vi "Main.vi"(11 "Module Admin":refnum<class "Delacor_lib_QMH_Cloneable Module Admin.lvclass">) -> ()   [LabVIEW 2020, in "Arduino stepper.lvlib"]
doc: "This template is based off of the Queued Message Handler design pattern and the Queued Message Handler project template that ships with LabVIEW.\n\nThe main difference is that the queue is private to this module and communication between modules is performed via Broadcast and Request events.\n\nRequest events are wrapped in public API methods and are handled in the Event Handling Loop (EHL) of this VI. Any module can register for Broadcast events sent by this module. The EHL generates messages based on user interface actions.\n\nThe Message Handling Loop (MHL) processes messages generated by the EHL, or by other messages. The messages are string values, so new messages can be added easily to the Message Cases case structure in the MHL. Each message cluster can also provide an optional value for Message Data, which is a variant that can be converted to whatever message-specific data is required.\n_____\nBased on DQMH Project Template 6.1.0.94."
uses:
  Arduino stepper.lvlib
  <vilib>/Delacor/Delacor QMH/Libraries/Cloneable Module Admin_class/Delacor_lib_QMH_Cloneable Module Admin.lvclass
  C:/Program Files (x86)/National Instruments/LabVIEW 2020/vi.lib/Delacor/Delacor QMH/Libraries/Module Admin_class/Delacor_lib_QMH_Module Admin.lvclass
  Module Data--cluster.ctl
  Stop continuous reading Argument--cluster.ctl
  <vilib>/Delacor/Delacor QMH/Libraries/Message Queue_class/Delacor_lib_QMH_Message Queue.lvclass/Delacor_lib_QMH_Message Queue.ctl
  <vilib>/Delacor/Delacor QMH/Libraries/Cloneable Module Admin_class/Delacor_lib_QMH_Cloneable Module Admin.lvclass/Delacor_lib_QMH_Cloneable Module Admin.ctl
  Stop Argument--cluster.ctl
  <vilib>/Delacor/Delacor QMH/Libraries/Module Admin_class/Delacor_lib_QMH_Module Admin.lvclass/Delacor_lib_QMH_Module Admin.ctl
  Connect Argument--cluster.ctl
  Support/COM params--typedef.ctl
  Connect (Reply Payload)--cluster.ctl
  Disconnect Argument--cluster.ctl
  Move motor Argument--cluster.ctl
  Support/Motor parameters.ctl
  Support/Motor direction -- enum.ctl
  Get position Argument--cluster.ctl
  Get position (Reply Payload)--cluster.ctl
  Read port continuously Argument--cluster.ctl
  Stop motor Argument--cluster.ctl
  Read end-stops Argument--cluster.ctl
  Read end-stops (Reply Payload)--cluster.ctl
  Read all info Argument--cluster.ctl
  <vilib>/Utility/miscctls.llb/LVPointTypeDef.ctl
  <vilib>/Instr/_visa.llb/VISA Flush IO Buffer Mask.ctl
  Support/Wake HL args--typedef.ctl
  <vilib>/Delacor/Delacor QMH/Libraries/Message Queue_class/Delacor_lib_QMH_Enqueue Message (Single).vi
  <vilib>/Delacor/Delacor QMH/Libraries/Cloneable Module Admin_class/Delacor_lib_QMH_Get Module ID.vi
  <vilib>/Delacor/Delacor QMH/Libraries/Module Admin_class/Delacor_lib_QMH_Get External Launch.vi
  <vilib>/Utility/error.llb/Error Cluster From Error Code.vi
  <vilib>/ErrorRing/Error Ring.xnode
  <vilib>/Delacor/Delacor QMH/Libraries/Message Queue_class/Delacor_lib_QMH_Message Queue.lvclass
panel:
  out "End-stops":cluster{"ES1":bool, "ES2":bool}
  out "read buffer 2":string
  out "Position":i32
  out "Data read":string
  out "*(type *) &x":string
  out "error out":errorcluster
  out "Status":string
  in  "Simulate EHL Error":bool
  in  "Simulate MHL Error":bool
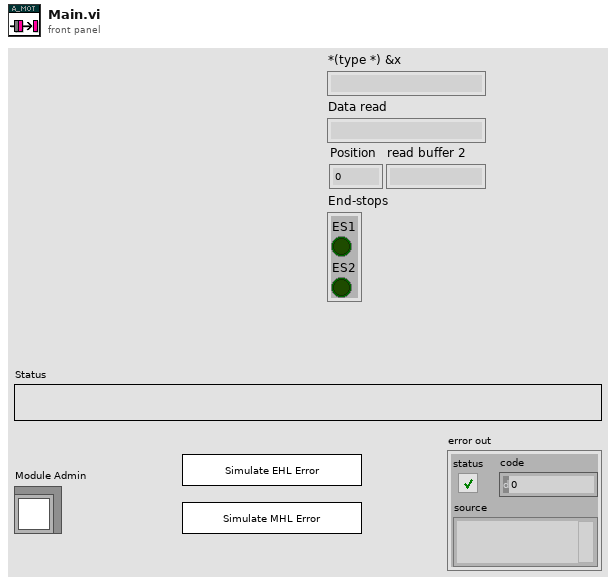
[diagram p1: front panel]
types:
  T1 = typedef "Arduino stepper.lvlib/Request Events--cluster.ctl" = cluster{"Stop Module":refnum<user-event>, "Show Panel":refnum<user-event>, "Hide Panel":refnum<user-event>, "Show Diagram":refnum<user-event>, "Get Module Execution Status":refnum<user-event>, "Connect":refnum<user-event>, "Disconnect":refnum<user-event>, "Move motor":refnum<user-event>, "Get position":refnum<user-event>, "Read port continuously":refnum<user-event>, "Stop continuous reading":refnum<user-event>, "Stop motor":refnum<user-event>, "Read end-stops":refnum<user-event>, "Read all info":refnum<user-event>}
  T2 = cluster{"Wake HL":refnum<user-event>, "Sleep HL":refnum<user-event>}
  T3 = typedef "Arduino stepper.lvlib/Module Data--cluster.ctl" = cluster{"Status":string, "VISA resource":refnum<visa-resource-name>, "Connected?":bool}
  T4 = typedef "Arduino stepper.lvlib/Stop continuous reading Argument--cluster.ctl" = cluster{"Module ID":i32, "Boolean":bool}
  T5 = enum32{"invalid lock state", "Not Locked", "Locked (No Password)", "Password-protected"}
  T6 = typedef "Arduino stepper.lvlib/Stop Argument--cluster.ctl" = cluster{"Module ID":i32, "Origin":string, "Exit via Stop Module Req?":bool, "Wait for Module to stop?":bool}
  T7 = typedef "Arduino stepper.lvlib/Connect Argument--cluster.ctl" = cluster{"Module ID":i32, "VISA resource":refnum<visa-resource-name>, "COM params":T8, "Wait Notifier":refnum<notifier>, "wait for reply":bool}
  T8 = typedef "Arduino stepper.lvlib/COM params--typedef.ctl" = cluster{"baud rate":u32, "data bits":u16, "parity":enum16{"None", "Odd", "Even", "Mark", "Space"}, "stop bits":u16, "flow control":u16}
  T9 = typedef "Arduino stepper.lvlib/Disconnect Argument--cluster.ctl" = cluster{"Module ID":i32, "Boolean":bool}
  T10 = typedef "Arduino stepper.lvlib/Move motor Argument--cluster.ctl" = cluster{"Module ID":i32, "Motor params":T11}
  T11 = typedef "Arduino stepper.lvlib/Motor parameters.ctl" = cluster{"Motor type":enum8{"", "Unipolar", "Bipolar"}, "Direction":T12, "Steps":u16, "Frequency (Hz)":u8, "Step type":enum8{"", "Half", "Full"}}
  T12 = typedef "Arduino stepper.lvlib/Motor direction -- enum.ctl" = enum8{"", "CW", "CCW"}
  T13 = typedef "Arduino stepper.lvlib/Get position Argument--cluster.ctl" = cluster{"Module ID":i32, "Wait Notifier":refnum<notifier>, "wait for reply":bool}
  T14 = typedef "Arduino stepper.lvlib/Read port continuously Argument--cluster.ctl" = cluster{"Module ID":i32, "Timeout":i32}
  T15 = typedef "Arduino stepper.lvlib/Stop motor Argument--cluster.ctl" = cluster{"Module ID":i32, "Boolean":bool}
  T16 = typedef "Arduino stepper.lvlib/Read end-stops Argument--cluster.ctl" = cluster{"Module ID":i32, "Wait Notifier":refnum<notifier>, "wait for reply":bool}
  T17 = typedef "Arduino stepper.lvlib/Read all info Argument--cluster.ctl" = cluster{"Module ID":i32, "Boolean":bool}
  T18 = typedef "LVPointTypeDef.ctl" = cluster{"Horizontal":i16, "Vertical":i16}
  T19 = enum32{"Invalid", "Standard", "Closed", "Hidden", "Minimized", "Maximized"}
  T20 = typedef "Arduino stepper.lvlib/Connect (Reply Payload)--cluster.ctl" = cluster{"error":errorcluster, "Connected?":bool}
  T21 = typedef "Arduino stepper.lvlib/Get position (Reply Payload)--cluster.ctl" = cluster{"Position":i32, "error":errorcluster, "End position?":bool}
  T22 = typedef "Arduino stepper.lvlib/Read end-stops (Reply Payload)--cluster.ctl" = cluster{"End-stops":cluster{"ES1":bool, "ES2":bool}, "error":errorcluster}
  T23 = typedef "Arduino stepper.lvlib/Wake HL args--typedef.ctl" = cluster{"VISA resource name":refnum<visa-resource-name>, "Timeout":i32, "Module ID":i32}
  T24 = typedef "VISA Flush IO Buffer Mask.ctl" = u16
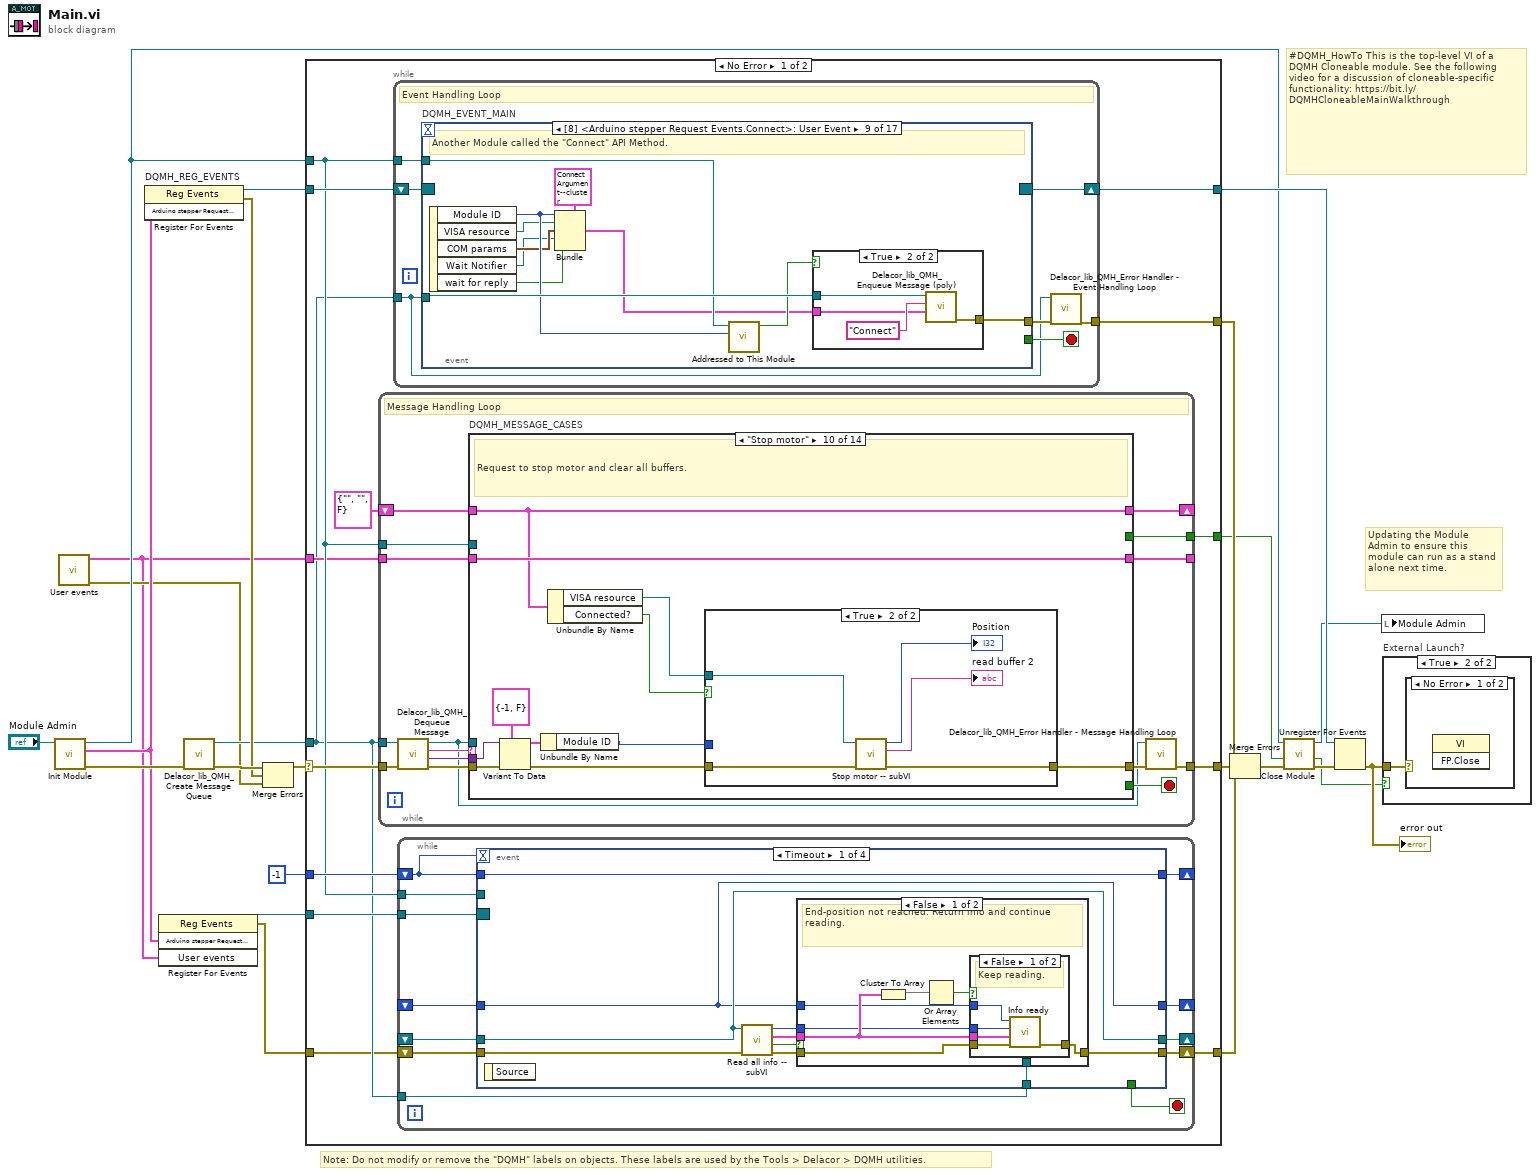
[diagram p0: block diagram]
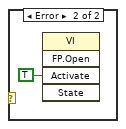
[diagram p3: hidden frame]
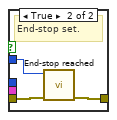
[diagram p4: hidden frame]
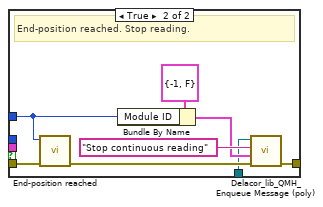
[diagram p5: hidden frame]
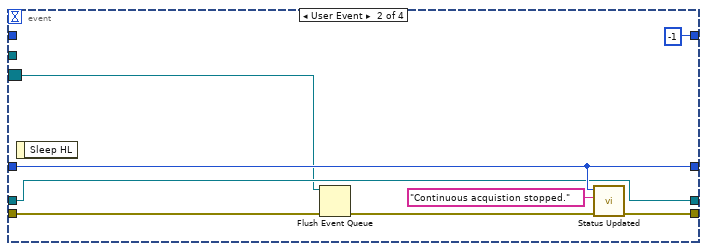
[diagram p6: hidden frame]
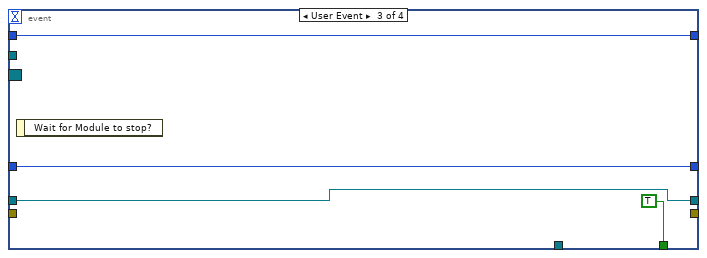
[diagram p7: hidden frame]
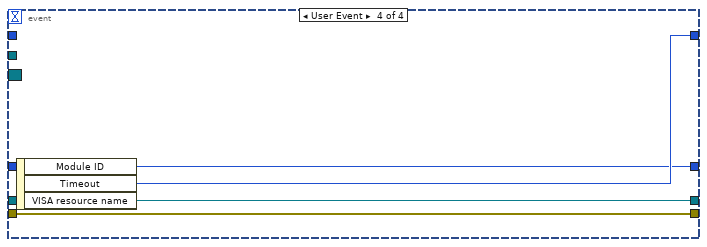
[diagram p8: hidden frame]
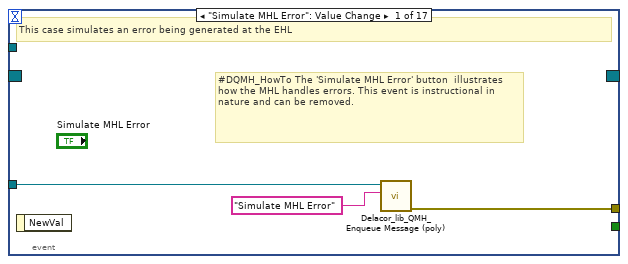
[diagram p9: hidden frame]
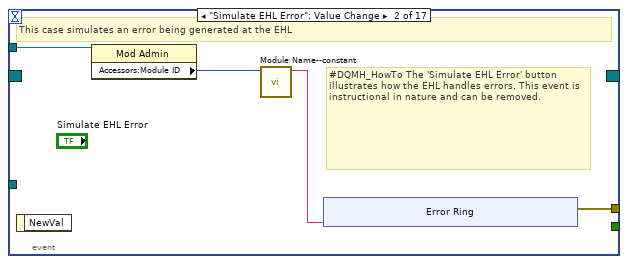
[diagram p10: hidden frame]
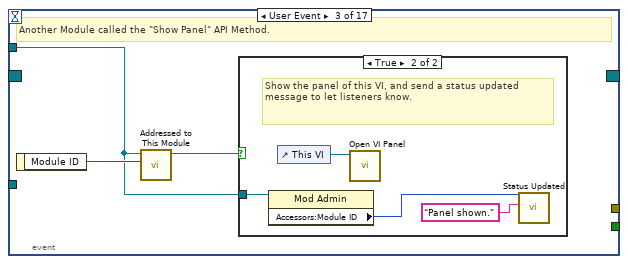
[diagram p11: hidden frame]
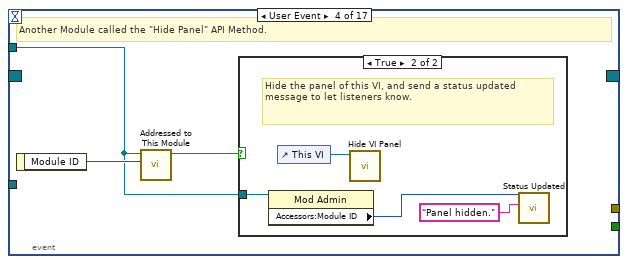
[diagram p13: hidden frame]
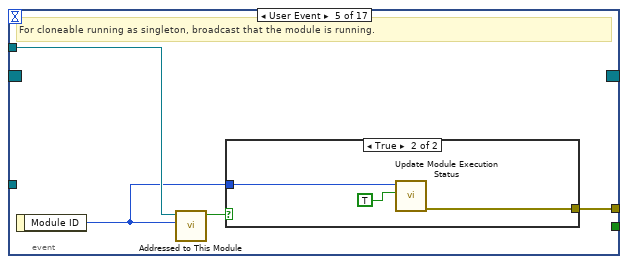
[diagram p15: hidden frame]
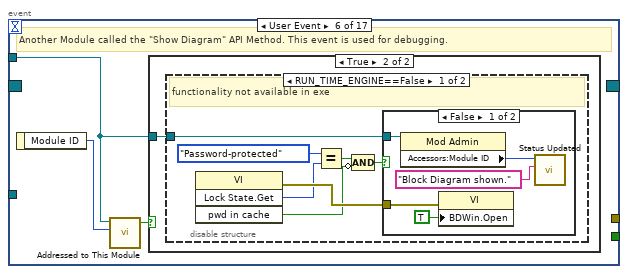
[diagram p17: hidden frame]
diagram:
  # "#DQMH_HowTo This is the top-level VI of a DQMH Cloneable module. See the following video for a discussion of cloneable-specific functionality: https://bit.ly/DQMHCloneableMainWalkthrough"
  # "Note: Do not modify or remove the \"DQMH\" labels on objects. These labels are used by the Tools > Delacor > DQMH utilities."
  # "Updating the Module Admin to ensure this module can run as a stand alone next time."
  n1 = call "Init Module.vi"("Cloneable Module Admin in"="Module Admin") -> ("error out"=w21:errorcluster, "Arduino stepper Request Events"=w8:T1, "Cloneable Module Admin out"=w5:refnum<class "Delacor_lib_QMH_Cloneable Module Admin.lvclass">)  [unwired: 8 in]
  n2 = call "User events.vi"() -> ("error out"=w4:errorcluster, "User events"=w3:T2)  [unwired: 10 in]
  n3 = register-events "DQMH_REG_EVENTS"(w8) -> (reference out=w14:refnum<event-registration>, error out=w16:errorcluster)  [unwired: 2 in]
  n4 = register-events(w8, w3) -> (reference out=w7:refnum<event-registration>, error out=w1:errorcluster)  [unwired: 2 in]
  n5 = call <vilib>:"Delacor_lib_QMH_Create Message Queue.vi"("error in"=w21) -> ("error out"=w18:errorcluster, "Message Queue"=w13:refnum<class "Delacor_lib_QMH_Message Queue.lvclass">)  [unwired: 9 in]
  n6 = Merge Errors(w18, w16, w4) -> (w17:errorcluster)
  n7 = case shown="No Error" w17 {
    selector: w17 -> [w36 w626]
    tunnel: [w38 w625] -> w22
    tunnel: [w35 w633] -> w15
    tunnel: w14 -> [w33 w633]
    tunnel: w13 -> [w27 w624]
    tunnel: [w37 _] -> w23
    tunnel: w5 -> [w29 w629]
    tunnel: [w32 _] -> w10
    tunnel: w7 -> [w31 _]
    tunnel: -1 -> [w30 _]
    tunnel: w3 -> [w28 _]
    tunnel: [w26 w623] -> w2
    tunnel: w1 -> [w25 w623]
    frame No Error {
      n8 = while {
        tunnel: w27 -> [w307]
        shift-right: [w311] -> _
        shift-left: T3 {"Status"="", "VISA resource"="", "Connected?"=FALSE} ("Data Cluster") -> [w312]
        tunnel: w36 -> [w315]
        tunnel: [w313] -> w38
        tunnel: w29 -> [w305]
        tunnel: [w304] -> w32
        tunnel: w28 -> [w303]
        tunnel: [w302] -> _
        stop <- w310 stop-if-true
        # "Message Handling Loop"
        n9 = call-dynamic "Delacor_lib_QMH_Dequeue Message.vi"("error in"=w315, "Message Queue in"=w307) -> ("error out"=w314:errorcluster, "Message Data"=w308:variant, "Message"=w309:string, "Message Queue out"=w306:refnum<class "Delacor_lib_QMH_Message Queue.lvclass">)  [unwired: 6 in]
        n10 = case "DQMH_MESSAGE_CASES" shown="\"Stop motor\"" w309 {
          selector: w309 -> [_ _ _ _ _ _ _ _ _ _ _ _ _ w610]
          tunnel: w306 -> [_ _ _ _ _ _ _ _ _ _ _ w566 w596 _]
          tunnel: w314 -> [w336 w359 w383 w409 w437 w469 w488 w511 w534 w551 w563 w575 w601 w612]
          tunnel: [w334 w351 w376 w403 w428 w460 w479 w507 w526 w543 w563 w571 w599 w613] -> w316
          tunnel: w312 -> [w327 w346 w373 w405 w427 w458 w482 w505 w533 w545 w562 w570 w584 w611]
          tunnel: [w326 w344 w371 w405 w427 w458 w482 w505 w533 w545 w562 w570 w584 w611] -> w311
          tunnel: [_ _ _ _ _ _ _ _ _ _ _ _ w595 _] -> w310
          tunnel: w308 -> [_ w357 w382 w408 w435 w467 w487 w510 w532 w550 _ w569 w593 _]
          tunnel: w305 -> [w321 _ _ _ _ _ _ _ w529 _ _ w568 w589 w608]
          tunnel: [_ _ _ _ _ _ _ _ _ _ _ _ w591 _] -> w304
          tunnel: w303 -> [w317 w347 w377 w402 w423 w459 w483 w502 w524 w546 w561 w564 w587 w606]
          tunnel: [w317 w347 w377 w402 w423 w459 w483 w502 w524 w546 w561 w564 w587 w606] -> w302
          frame "Initialize" {
            w318 = "Initial Message" ("Initial Message")
            # "#CodeNeeded - Initialize the appearance of the front panel."
            # "#CodeNeeded - Initialize your state data here."
            # "Initialize - Any operation that needs to be done before the module can receive messages. Synchronize Caller Events.vi will inform Start Module.vi that the module has launched and is ready to receive messages. Module Did Init.vi will broadcast that the module initialized."
            n11 = call "Synchronize Caller Events.vi"("error in (no error)"=w336, "Module Admin"=w321) -> ("error out"=w335:errorcluster, "Module Admin out"=w320:refnum<class "Delacor_lib_QMH_Cloneable Module Admin.lvclass">)  [unwired: 8 in]
            n12 = property class="Mod Admin"(reference=w320) -> ("Accessors:Module ID"=w323:i32, "Accessors:External Launch"=w322:bool)  [unwired: 1 in, 2 out]
            n13 = call "Module Name--constant.vi"("Module ID"=w323) -> ("Module Name"=w331:string)  [unwired: 10 in]
            n14 = property class="VI"("Front Panel.Title"=w331) -> (reference out=w333:refnum<vi>, error out=w338:errorcluster)  [unwired: 2 in]
            n15 = Select(t=T19."Hidden" ("State"), s=w322, f=T19."Standard" ("State")) -> (s? t:f=w328:T19)
            n16 = invoke class="VI" method="FP.Open"(reference=w333, error in=w338, "State"=w328) -> (reference out=w332:refnum<vi>, error out=w337:errorcluster)  [unwired: 2 in, 3 out]
            n17 = call "Module Name--constant.vi"("Module ID"=w323) -> ("Module Name"=w324:string)  [unwired: 10 in]
            n18 = Bundle By Name(cluster=w327, "Status"=w318) -> (w326:T3)
            n19 = invoke class="VI" method="FP.Center"(reference=w332, error in=w337) -> ()  [unwired: 1 in, 3 out]
            n20 = property on="Pane" class="Pane"("Origin"=T18 {"Horizontal"=0, "Vertical"=0}) -> ()  [unwired: 2 in, 2 out]
            n21 = call "Module Did Init.vi"("error in (no error)"=w335, "Initialized?"=TRUE, "Origin"=w324, "Module ID"=w323) -> ("error out"=w334:errorcluster)  [unwired: 7 in]
            "Status" <- w318
          }
          frame "Connect" {
            # "Request to connect to Arduino device using given communication parameters."
            n22 = Variant To Data(error in=w359, type=T7 {"Module ID"=-1, "VISA resource"="", "COM params"={"baud rate"=9600, "data bits"=8, "parity"=enum."None", "stop bits"=10, "flow control"=0}, "Wait Notifier"=refnum, "wait for reply"=FALSE} ("Connect Argument"), Variant=w357) -> (data=w350:T7, error out=w358:errorcluster)
            n23 = Unbundle By Name(w350) -> ("Module ID"=w342:i32, "COM params"=w349:T8, "VISA resource"=w348:refnum<visa-resource-name>, "Wait Notifier"=w355:refnum<notifier>, "wait for reply"=w354:bool)
            n24 = call "Connect and query.vi"("VISA resource"=w348, "COM params"=w349) -> ("error out"=w343:errorcluster, "String"=w339:string, "Connected?"=w341:bool, "VISA Refnum"=w345:refnum<visa-resource-name>)  [unwired: 6 in]
            n25 = case shown="False" w341 {
              tunnel: [w364 w368] -> w340
              tunnel: w343 -> [w362 w365]
              tunnel: w342 -> [w361 w366]
              tunnel: w339 -> [w360 _]
              frame False {
                n26 = call "Connection failed.vi"("error in"=w362, "String"=w360, "Connected?"=FALSE, "Module ID"=w361) -> ("error out"=w364:errorcluster)  [unwired: 7 in]
              }
              frame True {
                n27 = call "Device connected.vi"("error in"=w365, "Connected?"=TRUE, "Module ID"=w366) -> ("error out"=w368:errorcluster)  [unwired: 8 in]
              }
            }
            n28 = Bundle By Name(cluster=w346, "VISA resource"=w345, "Connected?"=w341) -> (w344:T3)
            n29 = Bundle By Name(cluster=T20 {"error"={"status"=FALSE, "code"=0, "source"=""}, "Connected?"=FALSE} ("Connect (Reply Payload)"), "Connected?"=w341, "error"=w340) -> (w353:T20)
            n30 = Merge Errors(w358, w340) -> (w351:errorcluster)
            n31 = case shown="True" w354 {
              tunnel: w355 -> [_ w370]
              tunnel: w353 -> [_ w369]
              frame False {
              }
              frame True {
                n32 = Send Notification(notification=w369, notifier=w370) -> ()  [unwired: 1 in, 2 out]
              }
            }
          }
          frame "Disconnect" {
            # "Request to disconnect from Arduino device."
            n33 = Variant To Data(error in=w383, type=T9 {"Module ID"=-1, "Boolean"=FALSE} ("Disconnect Argument"), Variant=w382) -> (data=w380:T9, error out=w378:errorcluster)
            n34 = Unbundle By Name(w373) -> ("VISA resource"=w379:refnum<visa-resource-name>, "Connected?"=w374:bool)
            n35 = Unbundle By Name(w380) -> ("Module ID"=w375:i32)
            n36 = case shown="True" w374 {
              tunnel: w379 -> [_ w394]
              tunnel: w378 -> [w384 w393]
              tunnel: [w384 w390] -> w376
              tunnel: w375 -> [_ w385]
              frame False {
              }
              frame True {
                w396 = T24 128 items=["Flush Receive Buffer"=16, "Write Transmit Buffer to Device"=32, "Flush Receive Buffer (No I/O)"=64, "Flush Transmit Buffer"=128] ("Mask")
                w397 = T24 64 items=["Flush Receive Buffer"=16, "Write Transmit Buffer to Device"=32, "Flush Receive Buffer (No I/O)"=64, "Flush Transmit Buffer"=128] ("Mask")
                n37 = Or(x=w397, y=w396) -> (x .or. y?=w395:T24)
                n38 = VISA Flush I/O Buffer(VISA resource name=w394, mask (16)=w395, error in (no error)=w393) -> (VISA resource name out=w392:refnum<visa-resource-name>, error out=w388:errorcluster)
                n39 = call "Wait ms.vi"("error in (no error)"=w388, "milliseconds to wait"=u32 100) -> ("error out"=w387:errorcluster)  [unwired: 9 in]
                n40 = VISA Close(VISA resource name=w392, error in (no error)=w387) -> (error out=w391:errorcluster)
                n41 = call "Device disconected.vi"("error in"=w391, "Connected?"=FALSE, "Module ID"=w385) -> ("error out"=w390:errorcluster)  [unwired: 8 in]
              }
            }
            n42 = Bundle By Name(cluster=w373, "Connected?"=FALSE) -> (w371:T3)
          }
          frame "Move motor" {
            # "Request to move the motor a certain number of steps."
            n43 = Variant To Data(error in=w409, type=T10 {"Module ID"=-1, "Motor params"={"Motor type"=enum."Unipolar", "Direction"=enum."CW", "Steps"=1000, "Frequency (Hz)"=20, "Step type"=enum."Full"}} ("Move motor Argument"), Variant=w408) -> (data=w401:T10, error out=w406:errorcluster)
            n44 = Unbundle By Name(w405) -> ("VISA resource"=w404:refnum<visa-resource-name>, "Connected?"=w399:bool)
            n45 = Unbundle By Name(w401) -> ("Module ID"=w398:i32, "Motor params"=w400:T11)
            n46 = case shown="True" w399 {
              tunnel: w406 -> [w412 w419]
              tunnel: w404 -> [_ w418]
              tunnel: [w413 w417] -> w403
              tunnel: w400 -> [_ w415]
              tunnel: w398 -> [w411 _]
              frame False {
                n47 = call "Status Updated.vi"("error in (no error)"=w412, "Status"="Device not connected. Cannot send commands. ", "Module ID"=w411) -> ("error out"=w413:errorcluster)  [unwired: 8 in]
              }
              frame True {
                n48 = call "Move motor--subVI.vi"("error in (no error)"=w419, "Motor params"=w415, "VISA Refnum in"=w418) -> ("error out"=w417:errorcluster, "Data read"=→"Data read":string, "Data written"=→"*(type *) &x":string)  [unwired: 6 in]
              }
            }
          }
          frame "Get position" {
            # "Request current position."
            n49 = Variant To Data(error in=w437, type=T13 {"Module ID"=-1, "Wait Notifier"=refnum, "wait for reply"=FALSE} ("Get position Argument"), Variant=w435) -> (data=w433:T13, error out=w436:errorcluster)
            n50 = Unbundle By Name(w427) -> ("VISA resource"=w426:refnum<visa-resource-name>, "Connected?"=w421:bool)
            n51 = Unbundle By Name(w433) -> ("Module ID"=w420:i32, "Wait Notifier"=w432:refnum<notifier>, "wait for reply"=w431:bool)
            n52 = case shown="True" w421 {
              tunnel: w426 -> [_ w446]
              tunnel: [w438 w441] -> w425
              tunnel: [_ w445] -> w424
              tunnel: [_ w442] -> w422
              tunnel: w420 -> [w439 w443]
              frame False {
                n53 = call "Status Updated.vi"("Status"="Device not connected. Cannot send commands. ", "Module ID"=w439) -> ("error out"=w438:errorcluster)  [unwired: 9 in]
              }
              frame True {
                n54 = call "Read position.vi"("VISA Refnum in"=w446) -> ("error out"=w444:errorcluster, "End position?"=w442:bool, "Position"=w445:i32)  [unwired: 8 in]
                n55 = case shown="True" w442 {
                  tunnel: w444 -> [w447 w450]
                  tunnel: w443 -> [_ w449]
                  tunnel: [w447 w448] -> w441
                  frame False {
                  }
                  frame True {
                    n56 = call "End-position reached.vi"("error in"=w450, "Module ID"=w449) -> ("error out"=w448:errorcluster)  [unwired: 9 in]
                  }
                }
              }
            }
            n57 = Bundle By Name(cluster=T21 {"Position"=0, "error"={"status"=FALSE, "code"=0, "source"=""}, "End position?"=FALSE} ("Get position (Reply Payload)"), "Position"=w424, "End position?"=w422, "error"=w425) -> (w430:T21)
            n58 = Merge Errors(w436, w425) -> (w428:errorcluster)
            n59 = case shown="True" w431 {
              tunnel: w432 -> [_ w452]
              tunnel: w430 -> [_ w451]
              frame False {
              }
              frame True {
                n60 = Send Notification(notification=w451, notifier=w452) -> ()  [unwired: 1 in, 2 out]
              }
            }
          }
          frame "Read end-stops" {
            # "Request to read end-stops from Arduino device."
            n61 = Variant To Data(error in=w469, type=T16 {"Module ID"=-1, "Wait Notifier"=refnum, "wait for reply"=FALSE} ("Read end-stops Argument"), Variant=w467) -> (data=w465:T16, error out=w468:errorcluster)
            n62 = Unbundle By Name(w458) -> ("VISA resource"=w457:refnum<visa-resource-name>, "Connected?"=w454:bool)
            n63 = Unbundle By Name(w465) -> ("Module ID"=w453:i32, "Wait Notifier"=w464:refnum<notifier>, "wait for reply"=w463:bool)
            n64 = case shown="True" w454 {
              tunnel: w457 -> [_ w475]
              tunnel: [_ w474] -> w456
              tunnel: [w470 w473] -> w455
              tunnel: w453 -> [w471 _]
              frame False {
                n65 = call "Status Updated.vi"("Status"="Device not connected. Cannot send commands. ", "Module ID"=w471) -> ("error out"=w470:errorcluster)  [unwired: 9 in]
              }
              frame True {
                n66 = call "Read end-stops -- subVI.vi"("VISA Refnum in"=w475) -> ("error out"=w473:errorcluster, "End-stops"=w474:cluster{"ES1":bool, "ES2":bool})  [unwired: 9 in]
                "End-stops" <- w474
              }
            }
            n67 = Merge Errors(w468, w455) -> (w460:errorcluster)
            n68 = Bundle By Name(cluster=T22 {"End-stops"={"ES1"=FALSE, "ES2"=FALSE}, "error"={"status"=FALSE, "code"=0, "source"=""}} ("Read end-stops (Reply Payload)"), "End-stops"=w456, "error"=w455) -> (w462:T22)
            n69 = case shown="True" w463 {
              tunnel: w464 -> [_ w477]
              tunnel: w462 -> [_ w476]
              frame False {
              }
              frame True {
                n70 = Send Notification(notification=w476, notifier=w477) -> ()  [unwired: 1 in, 2 out]
              }
            }
          }
          frame "Read all info" {
            # "Request to read position and end-stops in a single instruction."
            n71 = Variant To Data(error in=w488, type=T17 {"Module ID"=-1, "Boolean"=FALSE} ("Read all info Argument"), Variant=w487) -> (data=w485:T17, error out=w484:errorcluster)
            n72 = Unbundle By Name(w485) -> ("Module ID"=w480:i32)
            n73 = Unbundle By Name(w482) -> ("VISA resource"=w481:refnum<visa-resource-name>, "Connected?"=w478:bool)
            n74 = case shown="True" w478 {
              tunnel: w484 -> [_ w498]
              tunnel: w481 -> [_ w497]
              tunnel: w480 -> [w489 w495]
              tunnel: [w490 w492] -> w479
              frame False {
                n75 = call "Status Updated.vi"("Status"="Device not connected. Cannot send commands. ", "Module ID"=w489) -> ("error out"=w490:errorcluster)  [unwired: 9 in]
              }
              frame True {
                n76 = call "Read all info -- subVI.vi"("error in (no error)"=w498, "VISA Refnum in"=w497) -> ("error out"=w496:errorcluster, "End-stops"=w493:cluster{"ES1":bool, "ES2":bool}, "Position"=w494:i32)  [unwired: 6 in, 1 out]
                n77 = call "Info ready.vi"("error in"=w496, "End-stops"=w493, "Position"=w494, "Module ID"=w495) -> ("error out"=w492:errorcluster)  [unwired: 7 in]
              }
            }
          }
          frame "Read port continuously" {
            # "Request to wake up the helper loop for continuous monitoring of the serial port."
            n78 = Variant To Data(error in=w511, type=T14 {"Module ID"=-1, "Timeout"=-1} ("Wake HL Argument"), Variant=w510) -> (data=w508:T14, error out=w503:errorcluster)
            n79 = Unbundle By Name(w505) -> ("VISA resource"=w504:refnum<visa-resource-name>, "Connected?"=w499:bool)
            n80 = Unbundle By Name(w502) -> ("Wake HL"=w506:refnum<user-event>)
            n81 = Unbundle By Name(w508) -> ("Module ID"=w500:i32, "Timeout"=w501:i32)
            n82 = case shown="True" w499 {
              tunnel: [w512 w523] -> w507
              tunnel: w506 -> [_ w522]
              tunnel: w504 -> [_ w520]
              tunnel: w503 -> [w513 w521]
              tunnel: w501 -> [_ w516]
              tunnel: w500 -> [w514 w517]
              frame False {
                n83 = call "Status Updated.vi"("error in (no error)"=w513, "Status"="Device not connected. Cannot send commands. ", "Module ID"=w514) -> ("error out"=w512:errorcluster)  [unwired: 8 in]
              }
              frame True {
                n84 = Bundle By Name(cluster=T23 {"VISA resource name"="", "Timeout"=-1, "Module ID"=0} ("Wake HL"), "VISA resource name"=w520, "Module ID"=w517, "Timeout"=w516) -> (w518:T23)
                n85 = Generate User Event(user event=w522, event data cluster=w518, error in=w521) -> (error out=w523:errorcluster)  [unwired: 1 in, 1 out]
              }
            }
          }
          frame "Stop continuous reading" {
            # "Request to stop continuous reading of the serial port."
            n86 = Variant To Data(error in=w534, type=T4 {"Module ID"=-1, "Boolean"=FALSE} ("Stop continuous reading Argument"), Variant=w532) -> (data=w530:T4, error out=w527:errorcluster)
            n87 = Unbundle By Name(w530) -> ("Module ID"=w528:i32)  [unwired: 1 out]
            n88 = call "Addressed to This Module.vi"("Module ID from Argument"=w528, "Module Admin"=w529) -> ("Addressed to this instance?"=w525:bool)  [unwired: 8 in, 1 out]
            n89 = case shown="True" w525 {
              tunnel: w527 -> [w535 w540]
              tunnel: [w535 w539] -> w526
              tunnel: w524 -> [_ w538]
              frame False {
              }
              frame True {
                n90 = Unbundle By Name(w538) -> ("Sleep HL"=w537:refnum<user-event>)
                n91 = Generate User Event(user event=w537, event data cluster=FALSE ("event data"), error in=w540) -> (error out=w539:errorcluster)  [unwired: 1 in, 1 out]
              }
            }
          }
          frame "Stop motor" {
            # "Request to stop motor and clear all buffers."
            n92 = Variant To Data(error in=w551, type=T15 {"Module ID"=-1, "Boolean"=FALSE} ("Stop motor Argument"), Variant=w550) -> (data=w548:T15, error out=w547:errorcluster)
            n93 = Unbundle By Name(w548) -> ("Module ID"=w541:i32)
            n94 = Unbundle By Name(w545) -> ("VISA resource"=w544:refnum<visa-resource-name>, "Connected?"=w542:bool)
            n95 = case shown="True" w542 {
              tunnel: w547 -> [w553 w560]
              tunnel: w544 -> [_ w559]
              tunnel: [w554 w558] -> w543
              tunnel: w541 -> [w552 _]
              frame False {
                n96 = call "Status Updated.vi"("error in (no error)"=w553, "Status"="Device not connected. Cannot send commands. ", "Module ID"=w552) -> ("error out"=w554:errorcluster)  [unwired: 8 in]
              }
              frame True {
                n97 = call "Stop motor -- subVI.vi"("error in (no error)"=w560, "VISA Refnum in"=w559) -> ("error out"=w558:errorcluster, "read buffer 2"=→"read buffer 2":string, "Position"=→"Position":i32)  [unwired: 7 in]
              }
            }
          }
          frame "---Exit and Error Handling---" {
            # "Separator - the following cases handle errors and exit messages."
          }
          frame "Error" {
            # "#CodeRecommended - If you ever change the name of this \"Error\" message, you'll need to update the name in the Check Loop Error.vi as well."
            # "#CodeRecommended - If the module is running in standalone mode (External Launch = FALSE), this code will pop up an error dialog and call the 'Exit' message if an error occurs. Add more fine-grained error handling here."
            # "Error - Check the error message data and respond accordingly. This message is sent by the \"Error Handler\" VIs at the end of each loop in this application."
            n98 = property class="Mod Admin"(reference=w568) -> ("Accessors:External Launch"=w567:bool, "Accessors:Module ID"=w565:i32)  [unwired: 1 in, 2 out]
            n99 = Variant To Data(error in=w575, type=errorcluster {"status"=FALSE, "code"=0, "source"=""} ("error constant"), Variant=w569) -> (data=w576:errorcluster, error out=w573:errorcluster)
            n100 = call "Error Reported.vi"("Error"=w576, "Module ID"=w565) -> ()  [unwired: 9 in, 1 out]
            n101 = case shown="False" w567 {
              tunnel: [w581 _] -> w572
              tunnel: w566 -> [w579 _]
              tunnel: w576 -> [w580 _]
              frame False {
                # "If the module is running standalone, then pop up an error dialog and call the \"Exit\" message."
                n102 = call <vilib>:"Simple Error Handler.vi"("error in (no error)"=w580) -> ()  [unwired: 4 in, 5 out]
                n103 = call-poly <vilib>:"Delacor_lib_QMH_Enqueue Message (poly).vi"("Priority Message? (F)"=TRUE, "Message"="Exit", "Message Queue in"=w579) -> ("error out"=w581:errorcluster)  [unwired: 7 in, 1 out]
              }
              frame True {
                # "If the module was launched externally, calling the Error Reported broadcast VI is the only action performed by the \"Error\" message. The module's caller can then process the error appropriately."
              }
            }
            n104 = Merge Errors(w573, w572) -> (w571:errorcluster)
            n105 = local write "error out"(w571) -> ()
          }
          frame "Exit" {
            w594 = 91  # 91: not all Exit messages will have an argument
            w595 = TRUE  # Stop the VI
            # "Release the message queue reference"
            # "Exit - Exit the application."
            n106 = Variant To Data(error in=w601, type=T6 {"Module ID"=-1, "Origin"="", "Exit via Stop Module Req?"=FALSE, "Wait for Module to stop?"=FALSE} ("Stop Argument"), Variant=w593) -> (data=w590:T6, error out=w597:errorcluster)
            n107 = call <vilib>:"Clear Errors.vi"("error in (no error)"=w597, "specific error code to clear (0: all)"=w594) -> ("error out"=w600:errorcluster)  [unwired: 4 in, 1 out]
            n108 = Unbundle By Name(w584) -> ("VISA resource"=w583:refnum<visa-resource-name>, "Connected?"=w582:bool)
            n109 = call-dynamic "Delacor_lib_QMH_Release Message Queue.vi"("error in"=w600, "Message Queue"=w596) -> ("error out"=w586:errorcluster)  [unwired: 9 in]
            n110 = control-ref of="This VI"() -> (w588:refnum<vi>)
            n111 = call "Handle Exit.vi"("Stop Argument"=w590, "Module Admin in"=w589, "VI reference"=w588) -> ("error out"=w598:errorcluster, "Wait for Stop?"=w591:bool)  [unwired: 7 in]
            n112 = case shown="True" w582 {
              tunnel: w586 -> [w602 w605]
              tunnel: [w602 w604] -> w585
              tunnel: w583 -> [_ w603]
              frame False {
              }
              frame True {
                n113 = VISA Close(VISA resource name=w603, error in (no error)=w605) -> (error out=w604:errorcluster)
              }
            }
            n114 = Merge Errors(w585, w598) -> (w599:errorcluster)
          }
          frame Default {
            # "'Default' case only runs if there is a message that isn't defined in any of the other cases.  Output a programming error."
            n115 = property class="Mod Admin"(reference=w608) -> ("Accessors:Module ID"=w607:i32)  [unwired: 1 in, 2 out]
            n116 = call "Module Name--constant.vi"("Module ID"=w607) -> ("Module Name"=w609:string)  [unwired: 10 in]
            n117 = xnode "Error Ring"("parameter 0"=w610, "parameter 1"=w609) -> ("error out"=w614:errorcluster)
            n118 = Merge Errors(w612, w614) -> (w613:errorcluster)
          }
        }
        n119 = call-dynamic "Delacor_lib_QMH_Error Handler - Message Handling Loop.vi"("error in"=w316, "Message Queue in"=w306) -> ("dup error in"=w313:errorcluster)  [unwired: 8 in, 1 out]
      }
      n120 = while {
        tunnel: w27 -> [w100]
        shift-right: [w103] -> w35
        shift-left: w33 -> [w104]
        tunnel: [w105] -> w37
        tunnel: w29 -> [w101]
        stop <- w102 stop-if-true
        # "Event Handling Loop"
        n121 = event "DQMH_EVENT_MAIN" shown="[8] <Arduino stepper Request Events.Connect>: User Event" {
          selector: w104 -> [_ _ _ _ _ _ _ _ _ _ _ _ _ _ _ _ _]
          dyn-events: [_ _ _ _ _ _ _ _ _ _ _ _ _ _ _ _ _] -> w103
          timeout: _ -> [_ _ _ _ _ _ _ _ _ _ _ _ _ _ _ _ _]
          tunnel: [_ _ _ _ _ _ w161 _ _ _ _ _ _ _ _ _ _] -> w102
          tunnel: w100 -> [w108 _ _ _ _ _ w164 w180 w199 w211 w223 w236 w248 w260 w272 w285 w297]
          tunnel: [w109 w113 _ _ w138 _ w165 w183 w193 w204 w216 w228 w242 w253 w265 w277 w290] -> w106
          tunnel: w101 -> [_ w112 w121 w128 w136 w142 w163 w181 w197 w209 w221 w234 w246 w258 w270 w283 w295]
          event "Simulate MHL Error": Value Change {
            # "#DQMH_HowTo The 'Simulate MHL Error' button  illustrates how the MHL handles errors. This event is instructional in nature and can be removed."
            # "This case simulates an error being generated at the EHL"
            n122 = event-data() -> ()  [unwired: 1 in, 1 out]
            n123 = call-poly <vilib>:"Delacor_lib_QMH_Enqueue Message (poly).vi"("Message"="Simulate MHL Error", "Message Queue in"=w108) -> ("error out"=w109:errorcluster)  [unwired: 8 in, 1 out]
          }
          event "Simulate EHL Error": Value Change {
            # "#DQMH_HowTo The 'Simulate EHL Error' button  illustrates how the EHL handles errors. This event is instructional in nature and can be removed."
            # "This case simulates an error being generated at the EHL"
            n124 = event-data() -> ()  [unwired: 1 in, 1 out]
            n125 = property class="Mod Admin"(reference=w112) -> ("Accessors:Module ID"=w111:i32)  [unwired: 1 in, 2 out]
            n126 = call "Module Name--constant.vi"("Module ID"=w111) -> ("Module Name"=w110:string)  [unwired: 10 in]
            n127 = xnode "Error Ring"("parameter 0"=w110) -> ("error out"=w113:errorcluster)
          }
          event User Event {
            # "Another Module called the \"Show Panel\" API Method."
            n128 = event-data() -> ("Module ID"=w122:i32)  [unwired: 1 in]
            n129 = call "Addressed to This Module.vi"("Module ID from Argument"=w122, "Module Admin"=w121) -> ("Addressed to this instance?"=w123:bool)  [unwired: 8 in, 1 out]
            n130 = case shown="True" w123 {
              tunnel: w121 -> [_ w125]
              frame False {
              }
              frame True {
                # "Show the panel of this VI, and send a status updated message to let listeners know."
                n131 = property class="Mod Admin"(reference=w125) -> ("Accessors:Module ID"=w124:i32)  [unwired: 1 in, 2 out]
                n132 = control-ref of="This VI"() -> (w127:refnum<vi>)
                n133 = call "Open VI Panel.vi"("VI"=w127) -> ()  [unwired: 10 in, 1 out]
                n134 = call "Status Updated.vi"("Status"="Panel shown." ("format string"), "Module ID"=w124) -> ()  [unwired: 9 in, 1 out]
              }
            }
          }
          event User Event {
            # "Another Module called the \"Hide Panel\" API Method."
            n135 = event-data() -> ("Module ID"=w129:i32)  [unwired: 1 in]
            n136 = call "Addressed to This Module.vi"("Module ID from Argument"=w129, "Module Admin"=w128) -> ("Addressed to this instance?"=w130:bool)  [unwired: 8 in, 1 out]
            n137 = case shown="True" w130 {
              tunnel: w128 -> [_ w132]
              frame False {
              }
              frame True {
                # "Hide the panel of this VI, and send a status updated message to let listeners know."
                n138 = property class="Mod Admin"(reference=w132) -> ("Accessors:Module ID"=w131:i32)  [unwired: 1 in, 2 out]
                n139 = control-ref of="This VI"() -> (w134:refnum<vi>)
                n140 = call "Hide VI Panel.vi"("VI"=w134) -> ()  [unwired: 10 in, 1 out]
                n141 = call "Status Updated.vi"("Status"="Panel hidden." ("format string"), "Module ID"=w131) -> ()  [unwired: 9 in, 1 out]
              }
            }
          }
          event User Event {
            # "For cloneable running as singleton, broadcast that the module is running."
            n142 = event-data() -> ("Module ID"=w135:i32)  [unwired: 1 in]
            n143 = call "Addressed to This Module.vi"("Module ID from Argument"=w135, "Module Admin"=w136) -> ("Addressed to this instance?"=w137:bool)  [unwired: 8 in, 1 out]
            n144 = case shown="True" w137 {
              tunnel: [_ w141] -> w138
              tunnel: w135 -> [_ w140]
              frame False {
              }
              frame True {
                n145 = call "Update Module Execution Status.vi"("Running?"=TRUE, "Module ID"=w140) -> ("error out"=w141:errorcluster)  [unwired: 9 in]
              }
            }
          }
          event User Event {
            # "Another Module called the \"Show Diagram\" API Method. This event is used for debugging."
            n146 = event-data() -> ("Module ID"=w143:i32)  [unwired: 1 in]
            n147 = call "Addressed to This Module.vi"("Module ID from Argument"=w143, "Module Admin"=w142) -> ("Addressed to this instance?"=w144:bool)  [unwired: 8 in, 1 out]
            n148 = case shown="True" w144 {
              tunnel: w142 -> [_ w145]
              frame False {
              }
              frame True {
                n149 = disable-structure shown="RUN_TIME_ENGINE==False" {
                  disable-tunnel: w145 -> [w146 _]
                  frame condition #0 (active) {
                    # "functionality not available in exe"
                    n150 = invoke class="VI" method="Lock State.Get"() -> (error out=w152:errorcluster, "Get Lock State"=w151:T5, "pwd in cache"=w148:bool)  [unwired: 4 in, 1 out]
                    n151 = Equal?(x=T5."Password-protected", y=w151) -> (x = y?=w149:bool)
                    n152 = Compound Arithmetic op=AND(w149, invert w148) -> (w147:bool)
                    n153 = case shown="False" w147 {
                      tunnel: w152 -> [w157 _]
                      tunnel: w146 -> [w154 _]
                      frame False {
                        n154 = property class="Mod Admin"(reference=w154) -> ("Accessors:Module ID"=w153:i32)  [unwired: 1 in, 2 out]
                        n155 = property class="VI"(error in=w157, "BDWin.Open"=TRUE ("Block Diagram Window:Open")) -> ()  [unwired: 1 in, 2 out]
                        n156 = call "Status Updated.vi"("Status"="Block Diagram shown." ("format string"), "Module ID"=w153) -> ()  [unwired: 9 in, 1 out]
                      }
                      frame True {
                        # "Password-protected VI, and the password is not in the cache. Do not show the diagram."
                      }
                    }
                  }
                  frame condition #1 {
                  }
                }
              }
            }
          }
          event User Event {
            # "Another Module called the \"Stop Module\" API Method  or the Message Handling Loop below."
            n157 = event-data() -> ("Module ID"=w159:i32, "Wait for Module to stop?"=w160:bool, "Origin"=w158:string)  [unwired: 1 in]
            n158 = call "Addressed to This Module.vi"("Module ID from Argument"=w159, "Module Admin"=w163) -> ("Addressed to this instance?"=w162:bool)  [unwired: 8 in, 1 out]
            n159 = case shown="True" w162 {
              tunnel: [_ w177] -> w165
              tunnel: w164 -> [_ w173]
              tunnel: [_ TRUE] -> w161
              tunnel: w160 -> [_ w168]
              tunnel: w159 -> [_ w170]
              tunnel: w158 -> [_ w166]
              frame False {
              }
              frame True {
                # "The event can get fired from the Exit message. The queue gets destroyed there. In this case, the Enqueue VI will return error 1. It is safe to ignore, because the module is already exiting."
                n160 = local write "Status"(w166) -> ()
                n161 = Bundle By Name(cluster=T6 {"Module ID"=-1, "Origin"="", "Exit via Stop Module Req?"=FALSE, "Wait for Module to stop?"=FALSE} ("Stop Argument"), "Module ID"=w170, "Exit via Stop Module Req?"=TRUE, "Wait for Module to stop?"=w168) -> (w167:T6)
                n162 = call-poly <vilib>:"Delacor_lib_QMH_Enqueue Message (poly).vi"("Priority Message? (F)"=TRUE, "Message Data"=w167, "Message"="Exit", "Message Queue in"=w173) -> ("error out"=w178:errorcluster)  [unwired: 6 in, 1 out]
                n163 = call <vilib>:"Clear Errors.vi"("error in (no error)"=w178, "specific error code to clear (0: all)"=1) -> ("error out"=w177:errorcluster)  [unwired: 4 in, 1 out]
              }
            }
          }
          event Panel Close? {
            w182 = TRUE  # Discard the event, the MHL is responsible for closing and stopping this VI.
            # "Hide the panel or send the 'Exit' message if the user clicks the 'X' on the module main VI panel."
            n164 = event-data() -> ()  [unwired: 1 in, 1 out]
            n165 = property class="Mod Admin"(reference=w181) -> ("Accessors:External Launch"=w179:bool)  [unwired: 1 in, 2 out]
            n166 = case shown="True" w179 {
              tunnel: w180 -> [_ w187]
              tunnel: [_ w188] -> w183
              frame True {
                # "If externally launched, clicking the 'X' hides the panel, but doesn't close it."
                n167 = control-ref of="This VI"() -> (w184:refnum<vi>)
                n168 = call "Hide VI Panel.vi"("VI"=w184) -> ()  [unwired: 10 in, 1 out]
              }
              frame False {
                # "If run as a stand-alone VI, clicking the panel 'X' stops the VI."
                n169 = call-poly <vilib>:"Delacor_lib_QMH_Enqueue Message (poly).vi"("Priority Message? (F)"=TRUE, "Message"="Exit", "Message Queue in"=w187) -> ("error out"=w188:errorcluster)  [unwired: 7 in, 1 out]
              }
            }
            n170 = event-data("Discard?"=w182) -> ()  [unwired: 1 in, 1 out]
          }
          event User Event {
            # "Another Module called the \"Connect\" API Method."
            n171 = event-data() -> ("Module ID"=w194:i32, "VISA resource"=w192:refnum<visa-resource-name>, "COM params"=w191:T8, "Wait Notifier"=w190:refnum<notifier>, "wait for reply"=w189:bool)  [unwired: 1 in]
            n172 = Bundle(cluster=T7 {"Module ID"=-1, "VISA resource"="", "COM params"={"baud rate"=9600, "data bits"=8, "parity"=enum."None", "stop bits"=10, "flow control"=0}, "Wait Notifier"=refnum, "wait for reply"=FALSE} ("Connect Argument"), "Module ID"=w194, "VISA resource"=w192, "COM params"=w191, "Wait Notifier"=w190, "wait for reply"=w189) -> (w195:T7)
            n173 = call "Addressed to This Module.vi"("Module ID from Argument"=w194, "Module Admin"=w197) -> ("Addressed to this instance?"=w198:bool)  [unwired: 8 in, 1 out]
            n174 = case shown="True" w198 {
              tunnel: w199 -> [_ w203]
              tunnel: w195 -> [_ w201]
              tunnel: [_ w200] -> w193
              frame False {
              }
              frame True {
                n175 = call-poly <vilib>:"Delacor_lib_QMH_Enqueue Message (poly).vi"("Message Data"=w201, "Message"="Connect", "Message Queue in"=w203) -> ("error out"=w200:errorcluster)  [unwired: 7 in, 1 out]
              }
            }
          }
          event User Event {
            # "Another Module called the \"Disconnect\" API Method."
            n176 = event-data() -> ("Module ID"=w206:i32, "Boolean"=w205:bool)  [unwired: 1 in]
            n177 = Bundle(cluster=T9 {"Module ID"=-1, "Boolean"=FALSE} ("Disconnect Argument"), "Module ID"=w206, "Boolean"=w205) -> (w207:T9)
            n178 = call "Addressed to This Module.vi"("Module ID from Argument"=w206, "Module Admin"=w209) -> ("Addressed to this instance?"=w210:bool)  [unwired: 8 in, 1 out]
            n179 = case shown="True" w210 {
              tunnel: w211 -> [_ w215]
              tunnel: w207 -> [_ w213]
              tunnel: [_ w212] -> w204
              frame False {
              }
              frame True {
                n180 = call-poly <vilib>:"Delacor_lib_QMH_Enqueue Message (poly).vi"("Message Data"=w213, "Message"="Disconnect", "Message Queue in"=w215) -> ("error out"=w212:errorcluster)  [unwired: 7 in, 1 out]
              }
            }
          }
          event User Event {
            # "Another Module called the \"Move motor\" API Method."
            n181 = event-data() -> ("Module ID"=w218:i32, "Motor params"=w217:T11)  [unwired: 1 in]
            n182 = Bundle(cluster=T10 {"Module ID"=-1, "Motor params"={"Motor type"=enum."Unipolar", "Direction"=enum."CW", "Steps"=1000, "Frequency (Hz)"=20, "Step type"=enum."Full"}} ("Move motor Argument"), "Module ID"=w218, "Motor params"=w217) -> (w219:T10)
            n183 = call "Addressed to This Module.vi"("Module ID from Argument"=w218, "Module Admin"=w221) -> ("Addressed to this instance?"=w222:bool)  [unwired: 8 in, 1 out]
            n184 = case shown="True" w222 {
              tunnel: w223 -> [_ w227]
              tunnel: w219 -> [_ w225]
              tunnel: [_ w224] -> w216
              frame False {
              }
              frame True {
                n185 = call-poly <vilib>:"Delacor_lib_QMH_Enqueue Message (poly).vi"("Message Data"=w225, "Message"="Move motor", "Message Queue in"=w227) -> ("error out"=w224:errorcluster)  [unwired: 7 in, 1 out]
              }
            }
          }
          event User Event {
            # "Another Module called the \"Get position\" API Method."
            n186 = event-data() -> ("Module ID"=w231:i32, "Wait Notifier"=w230:refnum<notifier>, "wait for reply"=w229:bool)  [unwired: 1 in]
            n187 = Bundle(cluster=T13 {"Module ID"=-1, "Wait Notifier"=refnum, "wait for reply"=FALSE} ("Get position Argument"), "Module ID"=w231, "Wait Notifier"=w230, "wait for reply"=w229) -> (w232:T13)
            n188 = call "Addressed to This Module.vi"("Module ID from Argument"=w231, "Module Admin"=w234) -> ("Addressed to this instance?"=w235:bool)  [unwired: 8 in, 1 out]
            n189 = case shown="True" w235 {
              tunnel: w236 -> [_ w240]
              tunnel: w232 -> [_ w238]
              tunnel: [_ w237] -> w228
              frame False {
              }
              frame True {
                n190 = call-poly <vilib>:"Delacor_lib_QMH_Enqueue Message (poly).vi"("Message Data"=w238, "Message"="Get position", "Message Queue in"=w240) -> ("error out"=w237:errorcluster)  [unwired: 7 in, 1 out]
              }
            }
          }
          event User Event {
            # "Another Module called the \"Wake HL\" API Method."
            n191 = event-data() -> ("Module ID"=w243:i32, "Timeout"=w241:i32)  [unwired: 1 in]
            n192 = Bundle(cluster=T14 {"Module ID"=-1, "Timeout"=-1} ("Wake HL Argument"), "Module ID"=w243, "Timeout"=w241) -> (w244:T14)
            n193 = call "Addressed to This Module.vi"("Module ID from Argument"=w243, "Module Admin"=w246) -> ("Addressed to this instance?"=w247:bool)  [unwired: 8 in, 1 out]
            n194 = case shown="True" w247 {
              tunnel: w248 -> [_ w252]
              tunnel: w244 -> [_ w250]
              tunnel: [_ w249] -> w242
              frame False {
              }
              frame True {
                n195 = call-poly <vilib>:"Delacor_lib_QMH_Enqueue Message (poly).vi"("Message Data"=w250, "Message"="Read port continuously", "Message Queue in"=w252) -> ("error out"=w249:errorcluster)  [unwired: 7 in, 1 out]
              }
            }
          }
          event User Event {
            # "Another Module called the \"Stop continuous reading\" API Method."
            n196 = event-data() -> ("Module ID"=w255:i32, "Boolean"=w254:bool)  [unwired: 1 in]
            n197 = Bundle(cluster=T4 {"Module ID"=-1, "Boolean"=FALSE} ("Stop continuous reading Argument"), "Module ID"=w255, "Boolean"=w254) -> (w256:T4)
            n198 = call "Addressed to This Module.vi"("Module ID from Argument"=w255, "Module Admin"=w258) -> ("Addressed to this instance?"=w259:bool)  [unwired: 8 in, 1 out]
            n199 = case shown="True" w259 {
              tunnel: w260 -> [_ w264]
              tunnel: w256 -> [_ w262]
              tunnel: [_ w261] -> w253
              frame False {
              }
              frame True {
                n200 = call-poly <vilib>:"Delacor_lib_QMH_Enqueue Message (poly).vi"("Message Data"=w262, "Message"="Stop continuous reading", "Message Queue in"=w264) -> ("error out"=w261:errorcluster)  [unwired: 7 in, 1 out]
              }
            }
          }
          event User Event {
            # "Another Module called the \"Stop motor\" API Method."
            n201 = event-data() -> ("Module ID"=w267:i32, "Boolean"=w266:bool)  [unwired: 1 in]
            n202 = Bundle(cluster=T15 {"Module ID"=-1, "Boolean"=FALSE} ("Stop motor Argument"), "Module ID"=w267, "Boolean"=w266) -> (w268:T15)
            n203 = call "Addressed to This Module.vi"("Module ID from Argument"=w267, "Module Admin"=w270) -> ("Addressed to this instance?"=w271:bool)  [unwired: 8 in, 1 out]
            n204 = case shown="True" w271 {
              tunnel: w272 -> [_ w276]
              tunnel: w268 -> [_ w274]
              tunnel: [_ w273] -> w265
              frame False {
              }
              frame True {
                n205 = call-poly <vilib>:"Delacor_lib_QMH_Enqueue Message (poly).vi"("Message Data"=w274, "Message"="Stop motor", "Message Queue in"=w276) -> ("error out"=w273:errorcluster)  [unwired: 7 in, 1 out]
              }
            }
          }
          event User Event {
            # "Another Module called the \"Read end-stops\" API Method."
            n206 = event-data() -> ("Module ID"=w280:i32, "Wait Notifier"=w279:refnum<notifier>, "wait for reply"=w278:bool)  [unwired: 1 in]
            n207 = Bundle(cluster=T16 {"Module ID"=-1, "Wait Notifier"=refnum, "wait for reply"=FALSE} ("Read end-stops Argument"), "Module ID"=w280, "Wait Notifier"=w279, "wait for reply"=w278) -> (w281:T16)
            n208 = call "Addressed to This Module.vi"("Module ID from Argument"=w280, "Module Admin"=w283) -> ("Addressed to this instance?"=w284:bool)  [unwired: 8 in, 1 out]
            n209 = case shown="True" w284 {
              tunnel: w285 -> [_ w289]
              tunnel: w281 -> [_ w287]
              tunnel: [_ w286] -> w277
              frame False {
              }
              frame True {
                n210 = call-poly <vilib>:"Delacor_lib_QMH_Enqueue Message (poly).vi"("Message Data"=w287, "Message"="Read end-stops", "Message Queue in"=w289) -> ("error out"=w286:errorcluster)  [unwired: 7 in, 1 out]
              }
            }
          }
          event User Event {
            # "Another Module called the \"Read all info\" API Method."
            n211 = event-data() -> ("Module ID"=w292:i32, "Boolean"=w291:bool)  [unwired: 1 in]
            n212 = Bundle(cluster=T17 {"Module ID"=-1, "Boolean"=FALSE} ("Read all info Argument"), "Module ID"=w292, "Boolean"=w291) -> (w293:T17)
            n213 = call "Addressed to This Module.vi"("Module ID from Argument"=w292, "Module Admin"=w295) -> ("Addressed to this instance?"=w296:bool)  [unwired: 8 in, 1 out]
            n214 = case shown="True" w296 {
              tunnel: w297 -> [_ w301]
              tunnel: w293 -> [_ w299]
              tunnel: [_ w298] -> w290
              frame False {
              }
              frame True {
                n215 = call-poly <vilib>:"Delacor_lib_QMH_Enqueue Message (poly).vi"("Message Data"=w299, "Message"="Read all info", "Message Queue in"=w301) -> ("error out"=w298:errorcluster)  [unwired: 7 in, 1 out]
              }
            }
          }
        }
        n216 = call-dynamic "Delacor_lib_QMH_Error Handler - Event Handling Loop.vi"("error in"=w106, "Message Queue in"=w100) -> ("dup error in"=w105:errorcluster)  [unwired: 8 in, 1 out]
      }
      n217 = while {
        tunnel: w31 -> [w50]
        shift-right: [w48] -> _
        shift-left: w30 -> [w49]
        tunnel: w29 -> [w46]
        shift-right: [w45] -> _
        shift-left: _ -> [w44]
        shift-right: [w42] -> w26
        shift-left: w25 -> [w43]
        shift-right: [w41] -> _
        shift-left: _ -> [w40]
        tunnel: w27 -> [w39]
        stop <- w47 stop-if-true
        n218 = event shown="[0] Timeout" {
          selector: w50 -> [_ w84 _ _]
          dyn-events: _ -> [_ _ _ _]
          timeout: w49 -> [_ _ _ _]
          tunnel: w49 -> [w60 _ w95 _]
          tunnel: [w60 -1 ("Timeout") w95 w98] -> w48
          tunnel: [_ _ TRUE _] -> w47
          tunnel: w46 -> [_ _ _ _]
          tunnel: [w58 w87 w93 w97] -> w45
          tunnel: w44 -> [w58 w87 w93 _]
          tunnel: w43 -> [w59 w86 _ w99]
          tunnel: [w57 w90 _ w99] -> w42
          tunnel: [w56 w89 w92 w96] -> w41
          tunnel: w40 -> [w56 w89 w92 _]
          tunnel: w39 -> [w51 _ _ _]
          event Timeout {
            n219 = event-data() -> ()  [unwired: 1 in, 1 out]
            n220 = call "Read all info -- subVI.vi"("error in (no error)"=w59, "VISA Refnum in"=w58) -> ("error out"=w55:errorcluster, "End-position?"=w52:bool, "End-stops"=w54:cluster{"ES1":bool, "ES2":bool}, "Position"=w53:i32)  [unwired: 6 in]
            n221 = case shown="False" w52 {
              tunnel: w55 -> [w65 w79]
              tunnel: [w61 w80] -> w57
              tunnel: w56 -> [w62 w77]
              tunnel: w53 -> [w63 _]
              tunnel: w54 -> [w64 _]
              tunnel: w51 -> [_ w76]
              frame False {
                # "End-position not reached. Return info and continue reading."
                n222 = Cluster To Array(cluster=w64) -> (array=w67:bool[])
                n223 = Or Array Elements(Boolean array=w67) -> (logical OR=w66:bool)
                n224 = case shown="False" w66 {
                  tunnel: w65 -> [w72 w74]
                  tunnel: w64 -> [w71 _]
                  tunnel: w63 -> [w70 _]
                  tunnel: w62 -> [w69 w73]
                  tunnel: [w68 w75] -> w61
                  frame False {
                    # "Keep reading."
                    n225 = call "Info ready.vi"("error in"=w72, "End-stops"=w71, "Position"=w70, "Module ID"=w69) -> ("error out"=w68:errorcluster)  [unwired: 7 in]
                  }
                  frame True {
                    # "End-stop set."
                    n226 = call "End-stop reached.vi"("error in"=w74, "Module ID"=w73) -> ("error out"=w75:errorcluster)  [unwired: 9 in]
                  }
                }
              }
              frame True {
                # "End-position reached. Stop reading."
                n227 = call "End-position reached.vi"("error in"=w79, "Module ID"=w77) -> ("error out"=w78:errorcluster)  [unwired: 9 in]
                n228 = Bundle By Name(cluster=T4 {"Module ID"=-1, "Boolean"=FALSE} ("Stop continuous reading Argument"), "Module ID"=w77) -> (w81:T4)
                n229 = call-poly <vilib>:"Delacor_lib_QMH_Enqueue Message (poly).vi"("error in"=w78, "Message Data"=w81, "Message"="Stop continuous reading", "Message Queue in"=w76) -> ("error out"=w80:errorcluster)  [unwired: 6 in, 1 out]
              }
            }
          }
          event User Event {
            n230 = event-data() -> ()  [unwired: 1 in, 1 out]
            n231 = Flush Event Queue(0:w84, 3:w86) -> (11:w85:errorcluster)  [unwired: 4 in, 2 out]
            n232 = call "Status Updated.vi"("error in (no error)"=w85, "Status"="Continuous acquistion stopped.", "Module ID"=w89) -> ("error out"=w90:errorcluster)  [unwired: 8 in]
          }
          event User Event {
            n233 = event-data() -> ()  [unwired: 1 in, 1 out]
          }
          event User Event {
            n234 = event-data() -> ("Module ID"=w96:i32, "Timeout"=w98:i32, "VISA resource name"=w97:refnum<visa-resource-name>)  [unwired: 1 in]
          }
        }
      }
    }
    frame Error {
      n235 = call "Synchronize Caller Events.vi"("Module Admin"=w629) -> ("Module Admin out"=w628:refnum<class "Delacor_lib_QMH_Cloneable Module Admin.lvclass">)  [unwired: 9 in, 1 out]
      n236 = property class="Mod Admin"(reference=w628) -> ("Accessors:Module ID"=w627:i32)  [unwired: 1 in, 2 out]
      n237 = call-dynamic "Delacor_lib_QMH_Release Message Queue.vi"("error in"=w626, "Message Queue"=w624) -> ("error out"=w625:errorcluster)  [unwired: 9 in]
      n238 = call "Module Name--constant.vi"("Module ID"=w627) -> ("Module Name"=w632:string)  [unwired: 10 in]
      n239 = Format Into String(format string="An error occurred during initialization. %s is no longer running.", w632) -> (resulting string=w630:string)  [unwired: 2 in, 1 out]
      n240 = call "Error Reported.vi"("Additional Information"=w630, "Error"=w625, "Module ID"=w627) -> ()  [unwired: 8 in, 1 out]
    }
  }
  n241 = Merge Errors(w23, w22, w2) -> (w24:errorcluster)
  n242 = call "Close Module.vi"("error in"=w24, "Wait for stop?"=w10, "Module Admin in"=w5) -> ("error out"=w20:errorcluster, "External Launch"=w9:bool, "Module Admin out"=w11:refnum<class "Delacor_lib_QMH_Cloneable Module Admin.lvclass">)  [unwired: 6 in]
  n243 = Unregister For Events(event registration refnum=w15, error in=w20) -> (error out=w19:errorcluster)
  "error out" <- w19
  n244 = local write "Module Admin"(w11) -> ()
  n245 = case "External Launch?" shown="True" w9 {
    tunnel: w19 -> [_ w634]
    frame False {
    }
    frame True {
      n246 = case shown="No Error" w634 {
        frame No Error {
          n247 = invoke class="VI" method="FP.Close"() -> ()  [unwired: 3 in, 3 out]
        }
        frame Error {
          n248 = invoke class="VI" method="FP.Open"("Activate"=TRUE ("Activate?")) -> ()  [unwired: 4 in, 5 out]
        }
      }
    }
  }
